vi "Save IDE Options.vi"() -> ()   [LabVIEW 2020, in "Negentropic IDE.lvlib"]
uses:
  Negentropic IDE.lvlib
  IDE Options.ctl
panel:
  in  "IDE Options":T1
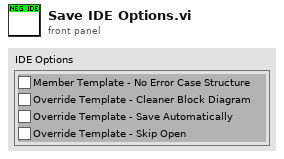
[diagram p1: front panel]
types:
  T1 = typedef "Negentropic IDE.lvlib/IDE Options.ctl" = cluster{"Member Template - No Error Case Structure":bool, "Override Template - Cleaner Block Diagram":bool, "Override Template - Save Automatically":bool, "Override Template - Skip Open":bool}
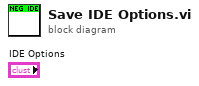
[diagram p0: block diagram]
diagram:
